vi "Initialize VIs Communication.vi"(8 "error in (no error)":errorcluster, 11 "Channel in":refnum<class "Channel.lvclass">) -> (0 "error out":errorcluster, 3 "Channel out":refnum<class "Channel.lvclass">)   [LabVIEW 2018, in "Channel.lvclass"]
doc: "Initialze the communcation with S4GUI"
uses:
  Channel.lvclass
  Channel.lvclass/Channel.ctl
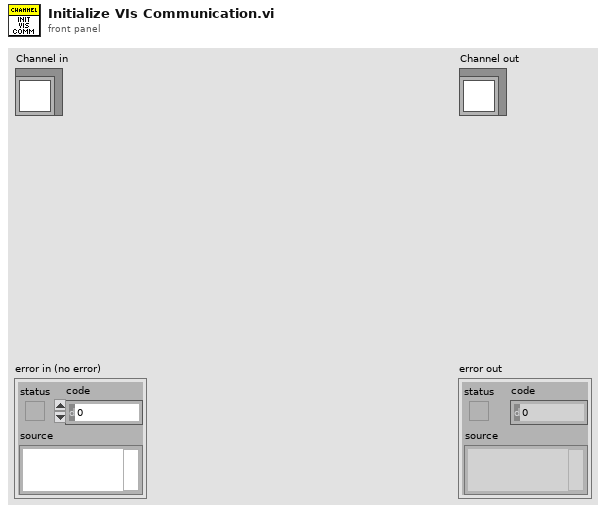
[diagram p1: front panel]
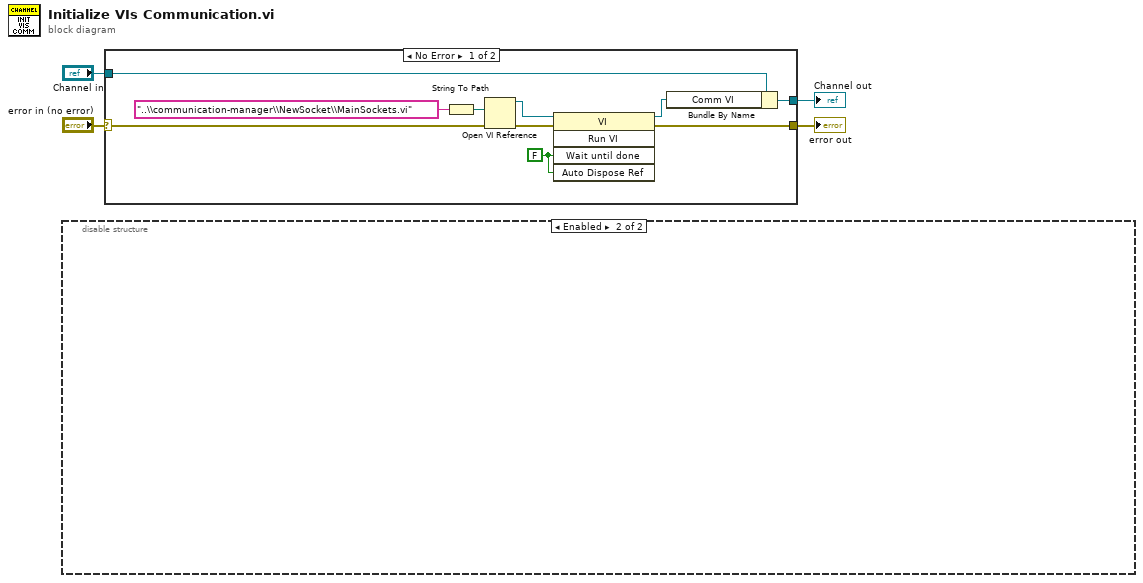
[diagram p0: block diagram]
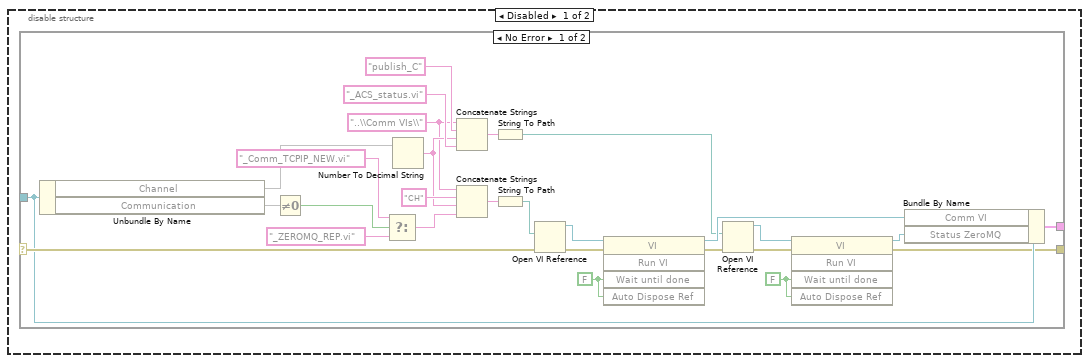
[diagram p2: hidden frame]
diagram:
  n1 = disable-structure shown="Enabled" {
    frame Disabled {
      n2 = case shown="No Error" {
        selector: _ -> [w27 w34]
        tunnel: [w14 w34] -> _
        tunnel: [w15 w33] -> _
        tunnel: _ -> [w23 w33]
        frame No Error {
          w5 = "..\\Comm VIs\\" ("name or relative path")
          w19 = FALSE ("Wait Until Done")
          w31 = FALSE ("Wait Until Done")
          n3 = Unbundle By Name(w23) -> ("Channel"=w10, "Communication"=w6)
          n4 = Not Equal To 0?(x=w6) -> (x != 0?=w7:bool)
          n5 = Select(t="_Comm_TCPIP_NEW.vi" ("name or relative path"), s=w7, f="_ZEROMQ_REP.vi" ("name or relative path")) -> (s? t:f=w25:string)
          n6 = Number To Decimal String(number=w10) -> (decimal integer string=w8:string)  [unwired: 1 in]
          n7 = Concatenate Strings(w5, "publish_C" ("name or relative path"), w8, "_ACS_status.vi" ("name or relative path")) -> (w11:string)
          n8 = Concatenate Strings(w5, "CH" ("name or relative path"), w8, w25) -> (w29:string)
          n9 = String To Path(string=w11) -> (path=w20:path)
          n10 = String To Path(string=w29) -> (path=w30:path)
          n11 = Open VI Reference(vi path=w30, error in (no error)=w27) -> (vi reference=w32:refnum<vi>, error out=w28:errorcluster)  [unwired: 4 in]
          n12 = invoke class="VI" method="Run VI"(reference=w32, error in=w28, "Wait until done"=w31, "Auto Dispose Ref"=w31) -> (reference out=w22:refnum<vi>, error out=w16:errorcluster)  [unwired: 1 in, 3 out]
          n13 = Open VI Reference(vi path=w20, error in (no error)=w16) -> (vi reference=w18:refnum<vi>, error out=w21:errorcluster)  [unwired: 4 in]
          n14 = invoke class="VI" method="Run VI"(reference=w18, error in=w21, "Wait until done"=w19, "Auto Dispose Ref"=w19) -> (reference out=w17:refnum<vi>, error out=w14:errorcluster)  [unwired: 1 in, 3 out]
          n15 = Bundle By Name(cluster=w23, "Comm VI"=w22, "Status ZeroMQ"=w17) -> (w15:cluster{})
        }
        frame Error {
        }
      }
    }
    frame Enabled {
    }
  }
  n16 = case shown="No Error" "error in (no error)" {
    selector: "error in (no error)" -> [w44 w46]
    tunnel: [w37 w46] -> w3
    tunnel: [w38 w45] -> w1
    tunnel: "Channel in" -> [w43 w45]
    frame No Error {
      w40 = FALSE ("Wait Until Done")
      n17 = String To Path(string="..\\communication-manager\\NewSocket\\MainSockets.vi" ("name or relative path")) -> (path=w41:path)
      n18 = Open VI Reference(vi path=w41, error in (no error)=w44) -> (vi reference=w39:refnum<vi>, error out=w42:errorcluster)  [unwired: 4 in]
      n19 = invoke class="VI" method="Run VI"(reference=w39, error in=w42, "Wait until done"=w40, "Auto Dispose Ref"=w40) -> (reference out=w35:refnum<vi>, error out=w37:errorcluster)  [unwired: 1 in, 3 out]
      n20 = Bundle By Name(cluster=w43, "Comm VI"=w35) -> (w38:refnum<class "Channel.lvclass">)
    }
    frame Error {
    }
  }
  "error out" <- w3
  "Channel out" <- w1
